vi "GetHighPrioritySensors.vi"() -> ()   [LabVIEW 2018]
uses:
  refnums.vi
  sensors.vi
panel:
  in  "Forward Position Wheel 4":dbl=0.75 format="%#_13g"
  in  "Forward Position Wheel 3":dbl=0.75 format="%#_13g"
  in  "Forward Position Wheel 2":dbl=0.75 format="%#_13g"
  in  "Forward Position Wheel 1":dbl=0.75 format="%#_13g"
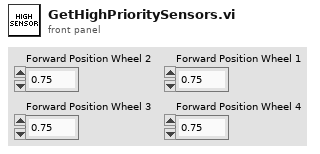
[diagram p1: front panel]
types:
  T1 = typedef "WPI_PotentiometerDevRef.ctl" = cluster{"DevStatus":errorcluster, "Analog Channel":T2, "Invert Output":bool}
  T2 = typedef "FPGA_AIChannel.ctl" = enum8{"AI 0", "AI 1", "AI 2", "AI 3", "AI MXP 0", "AI MXP 1", "AI MXP 2", "AI MXP 3", "Invalid"}
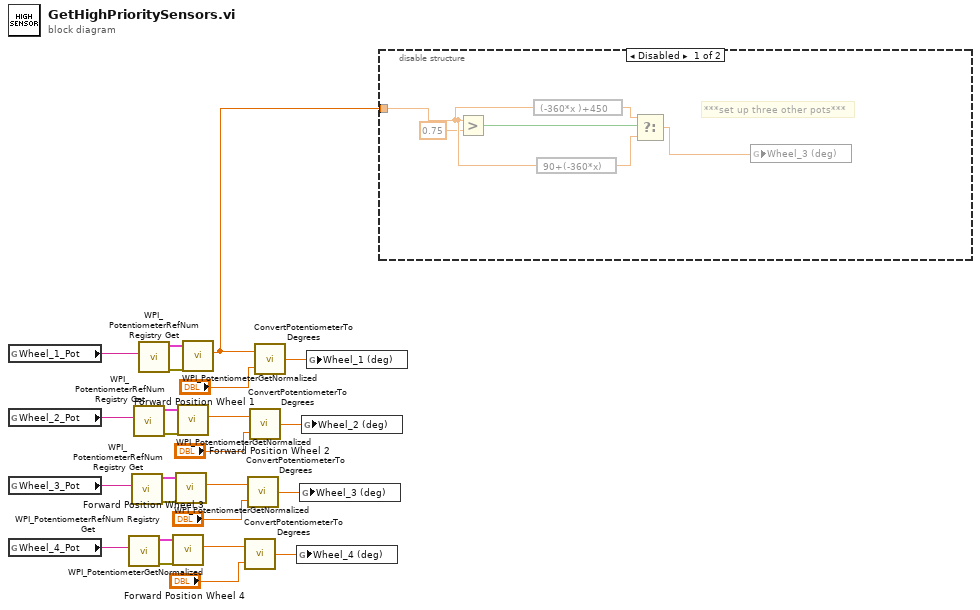
[diagram p0: block diagram]
diagram:
  n1 = global read "refnums.vi" "Wheel_1_Pot"() -> (w24:string)
  n2 = global read "refnums.vi" "Wheel_2_Pot"() -> (w18:string)
  n3 = global read "refnums.vi" "Wheel_3_Pot"() -> (w12:string)
  n4 = global read "refnums.vi" "Wheel_4_Pot"() -> (w6:string)
  n5 = call <vilib>:"WPI_PotentiometerRefNum Registry Get.vi"("refnum name"=w6) -> ("error out"=w5:errorcluster, "PotDevRef"=w4:T1)  [unwired: 9 in]
  n6 = call <vilib>:"WPI_PotentiometerRefNum Registry Get.vi"("refnum name"=w12) -> ("error out"=w11:errorcluster, "PotDevRef"=w10:T1)  [unwired: 9 in]
  n7 = call <vilib>:"WPI_PotentiometerRefNum Registry Get.vi"("refnum name"=w18) -> ("error out"=w17:errorcluster, "PotDevRef"=w16:T1)  [unwired: 9 in]
  n8 = call <vilib>:"WPI_PotentiometerRefNum Registry Get.vi"("refnum name"=w24) -> ("error out"=w23:errorcluster, "PotDevRef"=w22:T1)  [unwired: 9 in]
  n9 = call <vilib>:"WPI_PotentiometerGetNormalized.vi"("error in"=w5, "PotDevRef"=w4) -> ("Normalized Value"=w2:dbl)  [unwired: 7 in, 2 out]
  n10 = call <vilib>:"WPI_PotentiometerGetNormalized.vi"("error in"=w11, "PotDevRef"=w10) -> ("Normalized Value"=w8:dbl)  [unwired: 7 in, 2 out]
  n11 = call <vilib>:"WPI_PotentiometerGetNormalized.vi"("error in"=w17, "PotDevRef"=w16) -> ("Normalized Value"=w14:dbl)  [unwired: 7 in, 2 out]
  n12 = call <vilib>:"WPI_PotentiometerGetNormalized.vi"("error in"=w23, "PotDevRef"=w22) -> ("Normalized Value"=w20:dbl)  [unwired: 7 in, 2 out]
  n13 = call "ConvertPotentiometerToDegrees.vi"("Forward Position Wheel 1 [0-1]"="Forward Position Wheel 4", "Raw Potentiometer Value"=w2) -> ("Orientation (deg)"=w3:dbl)
  n14 = call "ConvertPotentiometerToDegrees.vi"("Forward Position Wheel 1 [0-1]"="Forward Position Wheel 3", "Raw Potentiometer Value"=w8) -> ("Orientation (deg)"=w9:dbl)
  n15 = call "ConvertPotentiometerToDegrees.vi"("Forward Position Wheel 1 [0-1]"="Forward Position Wheel 2", "Raw Potentiometer Value"=w14) -> ("Orientation (deg)"=w15:dbl)
  n16 = call "ConvertPotentiometerToDegrees.vi"("Forward Position Wheel 1 [0-1]"="Forward Position Wheel 1", "Raw Potentiometer Value"=w20) -> ("Orientation (deg)"=w21:dbl)
  n17 = global write "sensors.vi" "Wheel_4 (deg)"(w3) -> ()
  n18 = global write "sensors.vi" "Wheel_3 (deg)"(w9) -> ()
  n19 = global write "sensors.vi" "Wheel_2 (deg)"(w15) -> ()
  n20 = global write "sensors.vi" "Wheel_1 (deg)"(w21) -> ()
  n21 = disable-structure shown="Disabled" {
    disable-tunnel: w20 -> [w30 _]
    frame Disabled {
      # "***set up three other pots***"
      n22 = Greater?(x=w30, y=0.75) -> (0:w27:bool)
      n23 = expression code="(-360*x )+450" ("radians to degrees")(w30) -> (w28:dbl)
      n24 = expression code="90+(-360*x)" ("radians to degrees")(w30) -> (w29:dbl)
      n25 = Select(t=w28, s=w27, f=w29) -> (s? t:f=w25:dbl)
      n26 = global write "sensors.vi" "Wheel_3 (deg)"(w25) -> ()
    }
    frame Enabled {
    }
  }
